vi "Create Table.vi"(8 "error in (no error)":errorcluster) -> (0 "error out":errorcluster)   [LabVIEW 2020, in "Contabilidad.lvlib"]
uses:
  Contabilidad.lvlib
  <vilib>/drjdpowell/SQLite Library/SQL Connection/Open (path).vi
  <vilib>/drjdpowell/SQLite Library/SQL Connection/Open (string).vi
  <vilib>/AdvancedString/Path To Command Line String.vi
  <vilib>/drjdpowell/SQLite Library/SQL Connection/Execute SQL (No results).vi
  <vilib>/drjdpowell/SQLite Library/SQL Connection/Connection.lvclass
  <vilib>/drjdpowell/SQLite Library/SQLite.lvlib
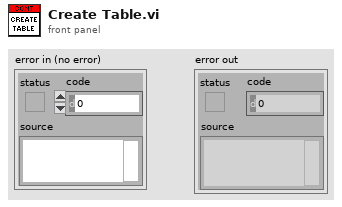
[diagram p1: front panel]
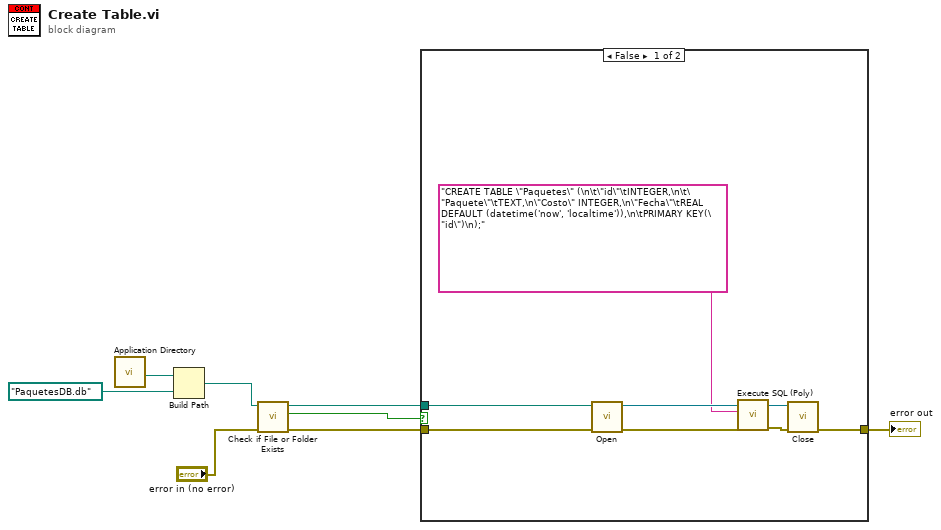
[diagram p0: block diagram]
diagram:
  n1 = call <vilib>:"Application Directory.vi"() -> ("Application Directory"=w3:path)
  n2 = Build Path(base path=w3, name or relative path=path "PaquetesDB.db") -> (appended path=w1:path)
  n3 = call <vilib>:"Check if File or Folder Exists.vi"("error in (no error)"="error in (no error)", "path"=w1) -> ("error out"=w4:errorcluster, "file or folder exists?"=w6:bool, "dup path"=w7:path)  [unwired: 7 in]
  n4 = case shown="False" w6 {
    tunnel: [w12 w17] -> w8
    tunnel: w7 -> [w9 _]
    tunnel: w4 -> [w10 w17]
    frame False {
      n5 = call-poly <vilib>:"Open.vi"("error in (no error)"=w10, "db file"=w9) -> ("error out"=w16:errorcluster, "SQLite Connection"=w15:refnum<class "Connection.lvclass">)  [unwired: 8 in]
      n6 = call-poly <vilib>:"Execute SQL (Poly).vi"("error in (no error)"=w16, "SQL"="CREATE TABLE \"Paquetes\" (\n\t\"id\"\tINTEGER,\n\t\"Paquete\"\tTEXT,\n\"Costo\" INTEGER,\n\"Fecha\"\tREAL DEFAULT (datetime('now', 'localtime')),\n\tPRIMARY KEY(\"id\")\n);", "SQLite Connection in"=w15) -> ("error out"=w14:errorcluster, "SQLite Connection"=w13:refnum<class "Connection.lvclass">)  [unwired: 7 in]
      n7 = call-dynamic "Close.vi"("error in (no error)"=w14, "SQLite Connection in"=w13) -> ("error out"=w12:errorcluster)  [unwired: 9 in]
    }
    frame True {
    }
  }
  "error out" <- w8
